vi "BASE_Reporting.vi"(8 "error in (no error)":errorcluster) -> (0 "error out":errorcluster)   [LabVIEW 2017]
uses:
  <vilib>/Utility/miscctls.llb/LVRangeTypeDef.ctl
  <vilib>/Utility/miscctls.llb/LVRowAndColumnTypeDef.ctl
  <vilib>/Utility/miscctls.llb/LVRowAndColumnUnsignedTypeDef.ctl
  <vilib>/addons/database/Connection.llb/DB Tools Open Connec (Path).vi
  <vilib>/Utility/file.llb/Write Delimited Spreadsheet (string).vi
  <vilib>/addons/database/NI_Database_API.lvlib
panel:
  in  "Machine Selection":string(combo)="ALL STATION"
  in  "Horizontal Slider Control":dbl(slide)=1.0 scale=0.0..19.0
  in  "Vertical Slider Control":dbl(slide)=1.0
  out "From Date":string
  out "appended path":path
  in  "SELECT FILTER":string(combo)="PART_NO"
  in  "Export to Excel":bool
  out "DESCRIPTION":string
  out "Data History Table":string[][](table)
  in  "TO DATE":timestamp format="%<%d/%m/%Y>T"
  in  "FROM DATE":timestamp format="%<%d/%m/%Y>T"
  in  "Back":bool
  in  "Show Report":bool
  # "BARCODE VERIFICATION SYSTEM REPORTS"
  # "Data History Table"
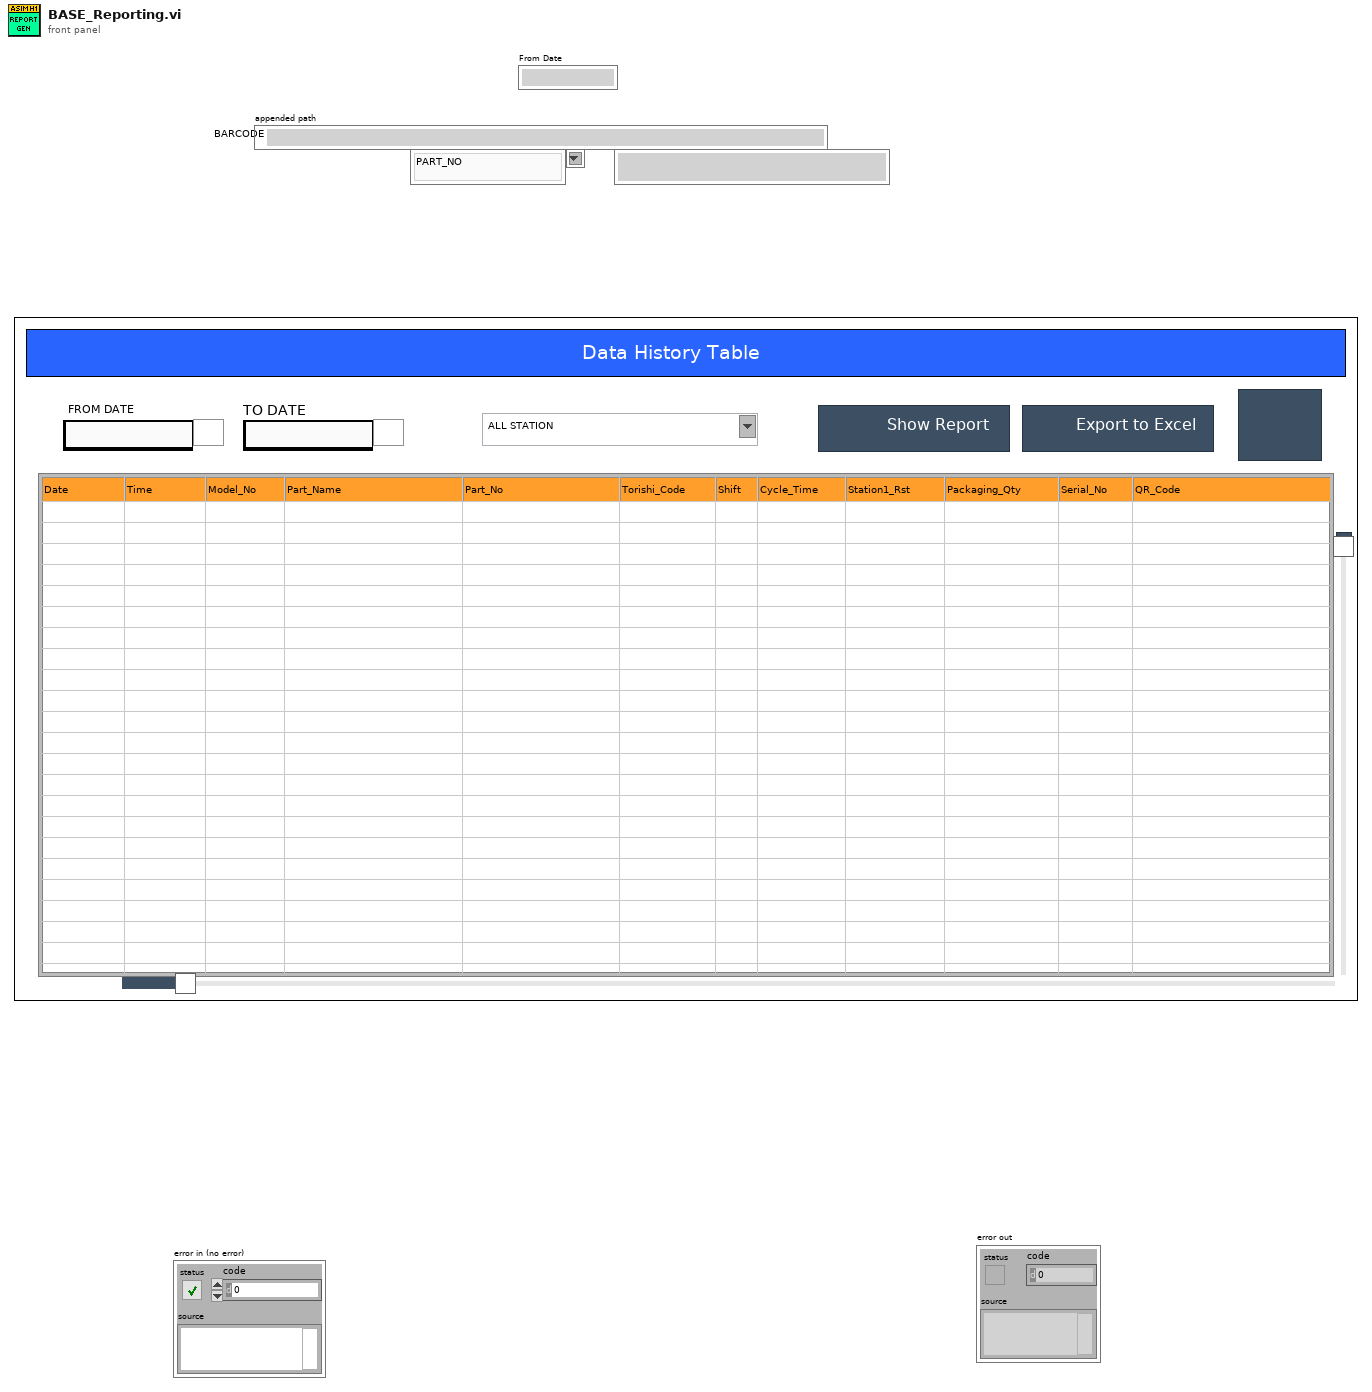
[diagram p1: front panel]
types:
  T1 = typedef "NI_Database_API.lvlib/Conn ObjectReference.ctl" = refnum<k1>
  T2 = typedef "LVRangeTypeDef.ctl" = cluster{"Minimum":dbl, "Maximum":dbl, "Increment":dbl, "Minor Increment":dbl, "Start":dbl}
  T3 = typedef "LVRowAndColumnTypeDef.ctl" = cluster{"Row":i32, "Column":i32}
  T4 = typedef "LVRowAndColumnUnsignedTypeDef.ctl" = cluster{"Row":u32, "Column":u32}
  T5 = enum32{"Invalid", "Standard", "Closed", "Hidden", "Minimized", "Maximized"}
  T6 = enum32{"invalid app kind", "Development System", "Run Time System", "Student Edition", "Embedded LabVIEW", "Evaluation", "Custom"}
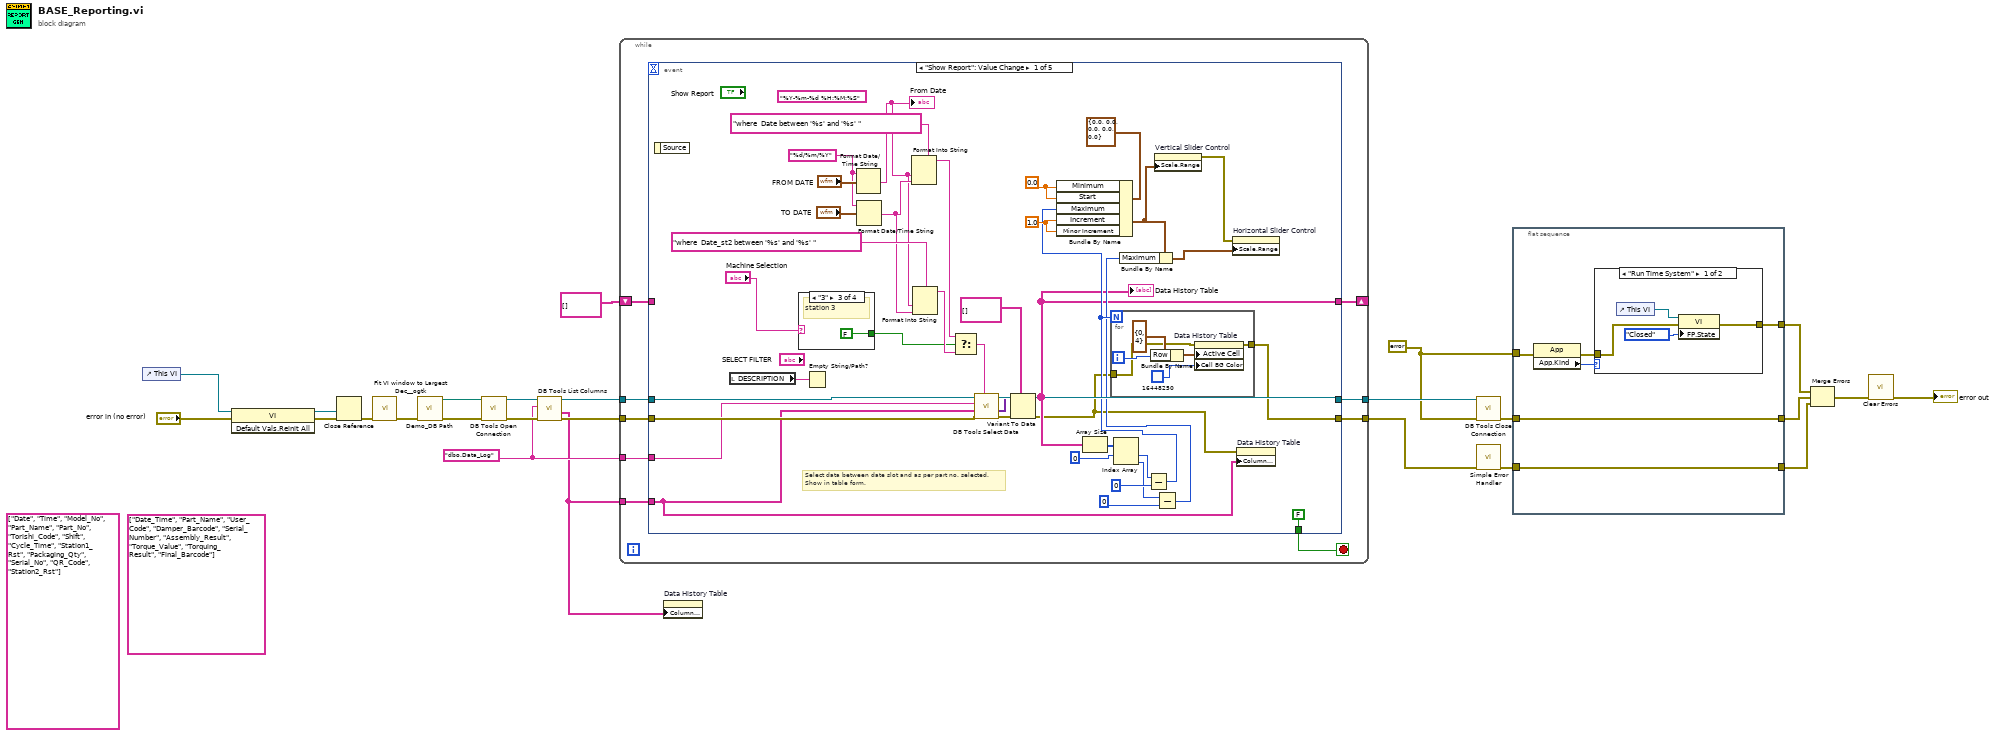
[diagram p0: block diagram]
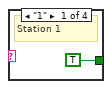
[diagram p3: hidden frame]
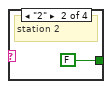
[diagram p4: hidden frame]
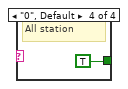
[diagram p5: hidden frame]
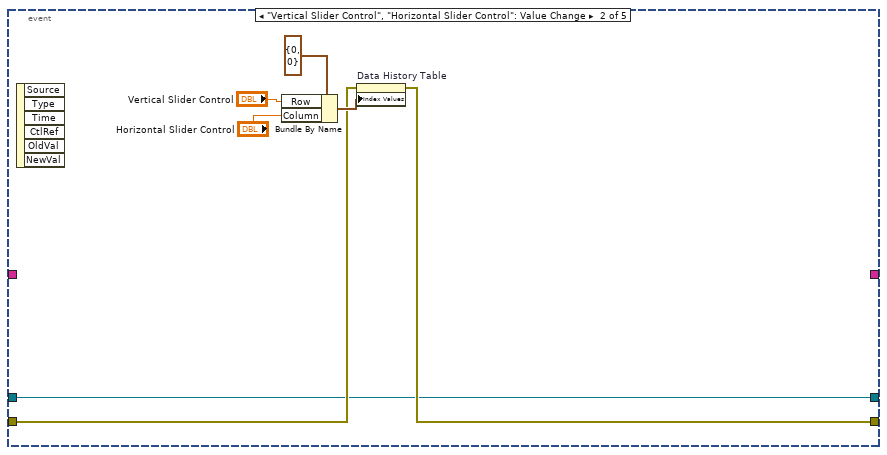
[diagram p6: hidden frame]
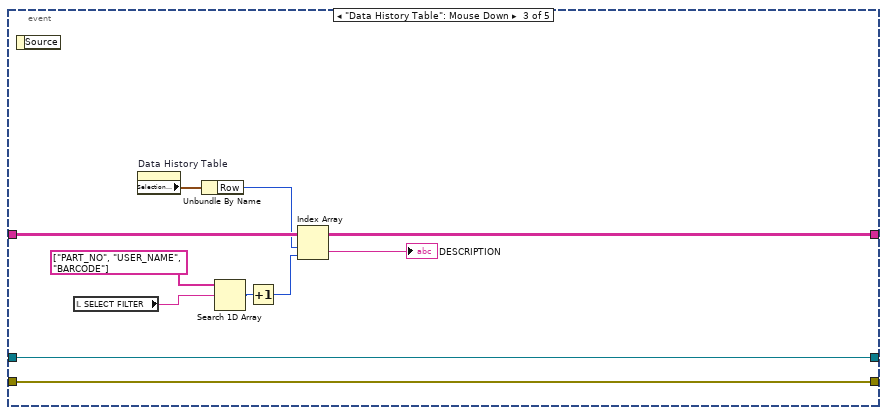
[diagram p7: hidden frame]
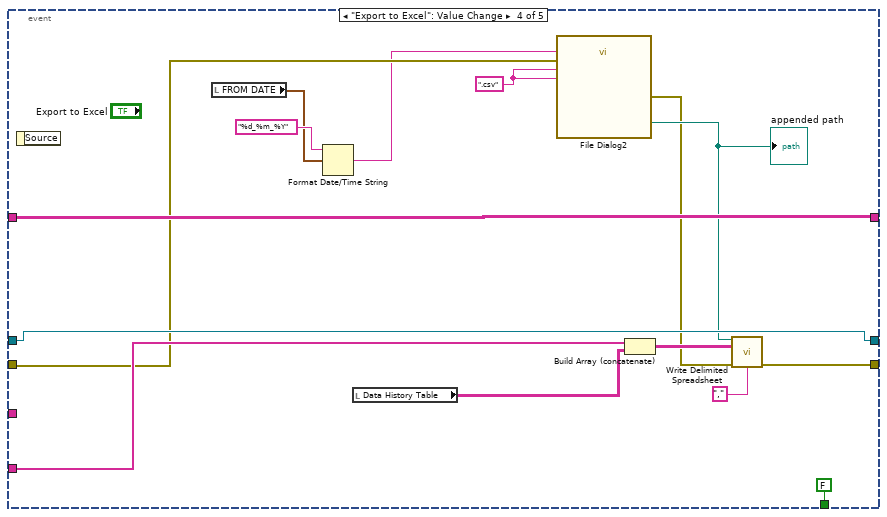
[diagram p8: hidden frame]
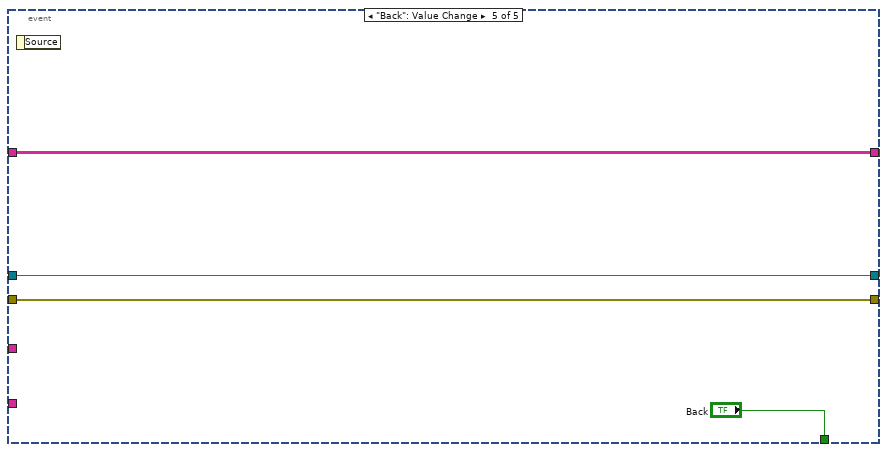
[diagram p9: hidden frame]
diagram:
  (unwired) string[] ["Date", "Time", "Model_No", "Part_Name", "Part_No", "Torishi_Code", "Shift", "Cycle_Time", "Station1_Rst", "Packaging_Qty", "Serial_No", "QR_Code", "Station2_Rst"] ("columns 2")
  w2 = "dbo.Data_Log" ("table")
  (unwired) string[] ["Date_Time", "Part_Name", "User_Code", "Damper_Barcode", "Serial_Number", "Assembly_Result", "Torque_Value", "Torquing_Result", "Final_Barcode"]
  w20 = errorcluster {"status"=FALSE, "code"=0, "source"=""} ("error in (no error)")
  n1 = control-ref of="This VI"() -> (w14:refnum<vi>)
  n2 = invoke class="VI" method="Default Vals.Reinit All"(reference=w14, error in="error in (no error)") -> (reference out=w12:refnum<vi>, error out=w11:errorcluster)  [unwired: 1 in, 1 out]
  n3 = Close Reference(reference=w12, error in (no error)=w11) -> (error out=w10:errorcluster)
  n4 = call <userlib>:"Fit VI window to Largest Dec__ogtk.vi"("error in (no error)"=w10) -> ("error out"=w3:errorcluster)  [unwired: 5 in, 1 out]
  n5 = call "Demo_DB Path.vi"("error in"=w3) -> ("error out"=w9:errorcluster, "DB Path"=w8:path)  [unwired: 9 in]
  n6 = call-poly <vilib>:"DB Tools Open Connection.vi"("error in (no error)"=w9, "connection information"=w8) -> ("error out"=w7:errorcluster, "connection reference"=w5:T1)  [unwired: 6 in]
  n7 = call <vilib>:"DB Tools List Columns.vi"("error in (no error)"=w7, "table"=w2, "connection reference"=w5) -> ("error out"=w6:errorcluster, "columns"=w1:string[], "connection reference out"=w4:T1)  [unwired: 1 in, 1 out]
  n8 = while {
    tunnel: w1 -> [w30]
    tunnel: w2 -> [w29]
    tunnel: w4 -> [w34]
    tunnel: [w31] -> w25
    tunnel: w6 -> [w33]
    tunnel: [w32] -> w23
    shift-right: [w27] -> _
    shift-left: string[][] [] -> [w26]
    stop <- w28 stop-if-true
    n9 = event shown="[0] \"Show Report\": Value Change" {
      selector: _ -> [_ _ _ _ _]
      dyn-events: _ -> [_ _ _ _ _]
      timeout: _ -> [_ _ _ _ _]
      tunnel: w34 -> [w73 w85 w97 w115 w118]
      tunnel: w33 -> [w72 w87 w96 w106 w117]
      tunnel: [w55 w86 w96 w110 w117] -> w32
      tunnel: [w71 w85 w97 w115 w118] -> w31
      tunnel: w30 -> [w41 _ _ w111 _]
      tunnel: w29 -> [w70 _ _ _ _]
      tunnel: [FALSE ("Back") _ _ FALSE ("Back") "Back"] -> w28
      tunnel: [w42 _ w100 w112 w116] -> w27
      tunnel: w26 -> [_ _ w100 w112 w116]
      event "Show Report": Value Change {
        w43 = 0.0 ("Start")
        w53 = 1.0 ("Increment")
        (unwired) "%Y-%m-%d %H:%M:%S"
        w60 = "%d/%m/%Y"
        # "Select data between date slot and as per part no. selected.\nShow in table form."
        n10 = event-data() -> ()  [unwired: 1 in, 1 out]
        n11 = local read "DESCRIPTION"() -> (w58:string)
        n12 = case shown="\"3\"" "Machine Selection" {
          tunnel: [TRUE FALSE FALSE TRUE] -> w35
          frame "1" {
            # "Station 1"
          }
          frame "2" {
            # "station 2"
          }
          frame "3" {
            # "station 3"
          }
          frame "0", Default {
            # "All station"
          }
        }
        n13 = Empty String/Path?(string/path=w58) -> ()  [unwired: 1 out]
        n14 = Format Date/Time String(time format string (%c)=w60, seconds (now)="FROM DATE") -> (date/time string=w37:string)  [unwired: 1 in]
        "From Date" <- w37
        n15 = Format Date/Time String(time format string (%c)=w60, seconds (now)="TO DATE") -> (date/time string=w38:string)  [unwired: 1 in]
        n16 = Format Into String(format string="where  Date between '%s' and '%s' ", w37, w38) -> (resulting string=w64:string)  [unwired: 2 in, 1 out]
        n17 = Format Into String(format string="where  Date_st2 between '%s' and '%s' ", w37, w38) -> (resulting string=w65:string)  [unwired: 2 in, 1 out]
        n18 = Select(t=w64, s=w35, f=w65) -> (s? t:f=w59:string)
        n19 = call <vilib>:"DB Tools Select Data.vi"("condition"=w59, "error in (no error)"=w72, "columns"=w41, "table"=w70, "connection reference"=w73) -> ("error out"=w66:errorcluster, "data"=w69:variant[][], "connection reference out"=w71:T1)  [unwired: 1 in]
        n20 = Variant To Data(error in=w66, type=string[][] [], Variant=w69) -> (data=w42:string[][], error out=w40:errorcluster)
        "Data History Table" <- w42
        n21 = Array Size(array=w42) -> (size(s)=w57:i32[])
        n22 = Index Array(array=w57, index #1=0 ("index")) -> (element #1=w48:i32, element #2=w45:i32)  [unwired: 1 in]
        n23 = Subtract(x=w48, y=0) -> (x-y=w47:i32)
        n24 = Bundle By Name(cluster=T2 {"Minimum"=0.0, "Maximum"=0.0, "Increment"=0.0, "Minor Increment"=0.0, "Start"=0.0} ("Scale.Range"), "Minimum"=w43, "Start"=w43, "Maximum"=w47, "Increment"=w53, "Minor Increment"=w53) -> (w52:T2)
        n25 = for {
          N: w47 -> [_]
          tunnel: w40 -> [w79]
          tunnel: [w78] -> w55
          i -> [w81]
          n26 = Bundle By Name(cluster=T3 {"Row"=0, "Column"=4} ("Active Cell:Active Cell"), "Row"=w81) -> (w82:T3)
          n27 = property on="Data History Table" class="Tbl (strict)"(error in=w79, "Active Cell"=w82, "Cell BG Color"=u32 16448250) -> (error out=w78:errorcluster)  [unwired: 1 in, 1 out]
        }
        n28 = property on="Vertical Slider Control" class="Slide (strict)"("Scale.Range"=w52) -> (error out=w50:errorcluster)  [unwired: 2 in, 1 out]
        n29 = Subtract(x=w45, y=0) -> (x-y=w46:i32)
        n30 = Bundle By Name(cluster=w52, "Maximum"=w46) -> (w51:T2)
        n31 = property on="Horizontal Slider Control" class="Slide (strict)"(error in=w50, "Scale.Range"=w51) -> ()  [unwired: 1 in, 2 out]
        n32 = property on="Data History Table" class="Tbl (strict)"(error in=w40, "Column Headers[]"=w41) -> ()  [unwired: 1 in, 2 out]
      }
      event "Vertical Slider Control", "Horizontal Slider Control": Value Change {
        n33 = event-data() -> ()  [unwired: 1 in, 6 out]
        n34 = Bundle By Name(cluster=T4 {"Row"=0, "Column"=0} ("Index Values"), "Row"="Vertical Slider Control", "Column"="Horizontal Slider Control") -> (w90:T4)
        n35 = property on="Data History Table" class="Tbl (strict)"(error in=w87, "Index Values"=w90) -> (error out=w86:errorcluster)  [unwired: 1 in, 1 out]
      }
      event "Data History Table": Mouse Down {
        n36 = event-data() -> ()  [unwired: 1 in, 1 out]
        n37 = local read "SELECT FILTER"() -> (w93:string)
        n38 = property on="Data History Table" class="Tbl (strict)"() -> ("Selection Start"=w99:T3)  [unwired: 2 in, 2 out]
        n39 = Unbundle By Name(w99) -> ("Row"=w98:i32)
        n40 = Search 1D Array(1D array=string[] ["PART_NO", "USER_NAME", "BARCODE"], element=w93) -> (index of element=w92:i32)  [unwired: 1 in]
        n41 = Increment(x=w92) -> (x+1=w91:i32)
        n42 = Index Array(array=w100, index (row)=w98, index (col)=w91) -> (element=→"DESCRIPTION":string)
      }
      event "Export to Excel": Value Change {
        w109 = ".csv" ("pattern label")
        n43 = event-data() -> ()  [unwired: 1 in, 1 out]
        n44 = local read "FROM DATE"() -> (w104:timestamp)
        n45 = Format Date/Time String(time format string (%c)="%d_%m_%Y", seconds (now)=w104) -> (date/time string=w103:string)  [unwired: 1 in]
        n46 = local read "Data History Table"() -> (w101:string[][])
        n47 = call "File Dialog2"("default name"=w103, "error in"=w106, "pattern (all files)"=w109, "pattern label"=w109) -> ("selected path"=w108:path, "error out"=w107:errorcluster)  [unwired: 8 in, 2 out]
        "appended path" <- w108
        n48 = Build Array (concatenate)(w111, w101) -> (w113:string[][])
        n49 = call-poly <vilib>:"Write Delimited Spreadsheet.vi"("file path (dialog if empty)"=w108, "2D data"=w113, "error in (no error)"=w107, "delimiter (\\t)"="," ("delimiter (\\t)")) -> ("error out"=w110:errorcluster)  [unwired: 10 in, 1 out]
      }
      event "Back": Value Change {
        n50 = event-data() -> ()  [unwired: 1 in, 1 out]
      }
    }
  }
  n51 = property on="Data History Table" class="Tbl (strict)"("Column Headers[]"=w1) -> ()  [unwired: 2 in, 2 out]
  n52 = call <vilib>:"DB Tools Close Connection.vi"("error in (no error)"=w20, "connection reference"=w25) -> ("error out"=w18:errorcluster)  [unwired: 5 in]
  n53 = call <vilib>:"Simple Error Handler.vi"("error in (no error)"=w23) -> ("error out"=w16:errorcluster)  [unwired: 4 in, 4 out]
  n54 = flat-sequence {
    tunnel: [w123] -> w21
    tunnel: w20 -> [w122]
    tunnel: [w121] -> w19
    tunnel: w18 -> [w121]
    tunnel: [w120] -> w17
    tunnel: w16 -> [w120]
    frame #0 {
      n55 = property class="App"(error in=w122) -> (error out=w124:errorcluster, "App.Kind"=w125:T6)  [unwired: 1 in, 1 out]
      n56 = case shown="\"Run Time System\"" w125 {
        tunnel: w124 -> [w127 w130]
        tunnel: [w126 w130] -> w123
        frame "Run Time System" {
          n57 = control-ref of="This VI"() -> (w129:refnum<vi>)
          n58 = property class="VI"(reference=w129, error in=w127, "FP.State"=T5."Closed" ("Front Panel Window:State")) -> (error out=w126:errorcluster)  [unwired: 1 out]
        }
        frame "Development System", Default {
        }
      }
    }
  }
  n59 = Merge Errors(w21, w19, w17) -> (w22:errorcluster)
  n60 = call <vilib>:"Clear Errors.vi"("error in (no error)"=w22) -> ("error out"=→"error out":errorcluster)  [unwired: 5 in, 1 out]
